vi "Update Dates.vi"(9 "date time rec":T1, 10 "Display State In":cluster{"Month":i32, "Day":i32, "Year":i32}, 11 "Dates":refnum<vi>) -> ()   [LabVIEW 2019, in "Custom Calendar.xctl"]
uses:
  Custom Calendar.xctl
panel:
  out "Month":string[][](array[string])
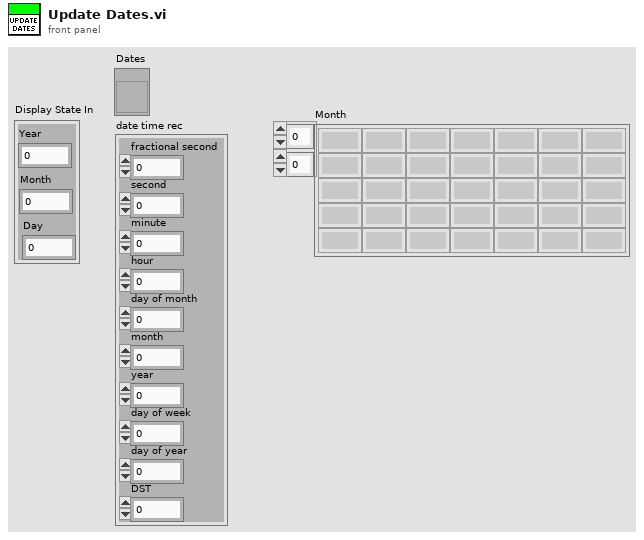
[diagram p1: front panel]
types:
  T1 = cluster{"fractional second":dbl, "second":i32, "minute":i32, "hour":i32, "day of month":i32, "month":i32, "year":i32, "day of week":i32, "day of year":i32, "DST":i32}
  T2 = typedef "LVDateTimeRec.ctl" = cluster{"fractional second":dbl, "second":i32, "minute":i32, "hour":i32, "day of month":i32, "month":i32, "year":i32, "day of week":i32, "day of year":i32, "DST":i32}
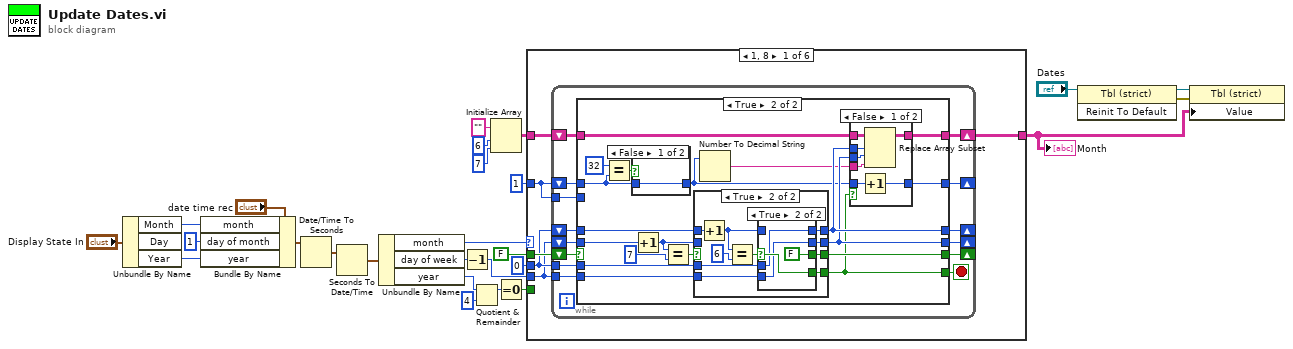
[diagram p0: block diagram]
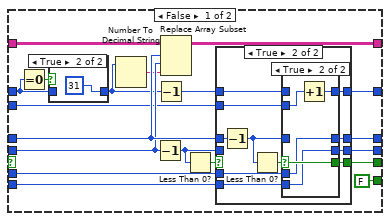
[diagram p2: hidden frame]
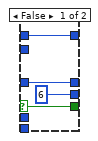
[diagram p5: hidden frame]
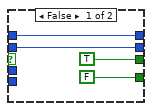
[diagram p7: hidden frame]
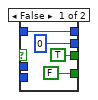
[diagram p8: hidden frame]
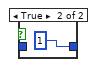
[diagram p9: hidden frame]
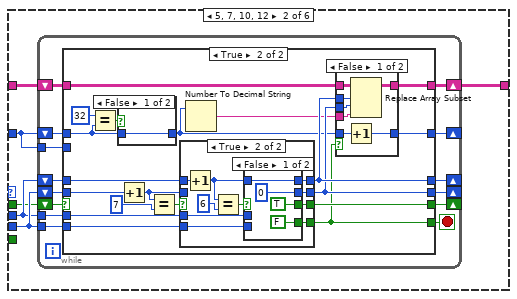
[diagram p10: hidden frame]
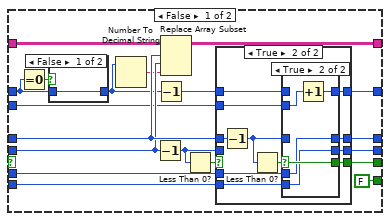
[diagram p11: hidden frame]
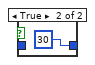
[diagram p12: hidden frame]
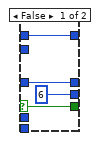
[diagram p14: hidden frame]
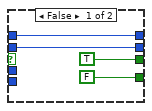
[diagram p16: hidden frame]
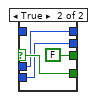
[diagram p17: hidden frame]
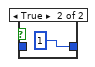
[diagram p18: hidden frame]
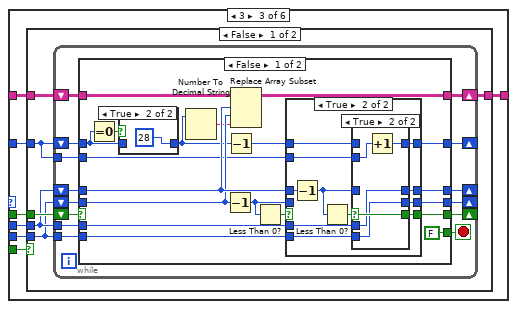
[diagram p19: hidden frame]
diagram:
  n1 = Unbundle By Name("Display State In") -> ("Month"=w14:i32, "Year"=w15:i32)  [unwired: 1 out]
  n2 = Bundle By Name(cluster="date time rec", "month"=w14, "day of month"=1, "year"=w15) -> (w26:T1)
  n3 = Date/Time To Seconds(2:w26) -> (0:w25:timestamp)  [unwired: 1 in]
  n4 = Seconds To Date/Time(time stamp (now)=w25) -> (date time rec=w23:T2)  [unwired: 1 in]
  n5 = Unbundle By Name(w23) -> ("month"=w22:i32, "day of week"=w8:i32, "year"=w20:i32)
  n6 = Decrement(x=w8) -> (x-1=w9:i32)
  n7 = Quotient & Remainder(x=w20, y=4) -> (x-y*floor(x/y)=w18:i32)  [unwired: 1 out]
  n8 = Initialize Array("", 6 ("dimension size"), 7 ("dimension size")) -> (w10:string[][])
  n9 = Equal To 0?(x=w18) -> (x = 0?=w17:bool)
  n10 = case shown="1, 8" w22 {
    tunnel: 1 ("day of month") -> [w27 w145 w265 w507 w747 _]
    tunnel: w10 -> [w32 w149 w266 w506 w748 w860]
    tunnel: [w31 w148 w261 w502 w743 w860] -> w1
    tunnel: w9 -> [w28 w147 w262 w503 w744 _]
    tunnel: 0 -> [w29 w146 w263 w504 w746 _]
    tunnel: FALSE -> [w30 w144 w264 w505 w745 _]
    tunnel: w17 -> [_ _ w267 w508 _ _]
    frame 1, 8 {
      n11 = while {
        shift-right: [w38] -> _
        shift-left: w29 -> [w46]
        shift-right: [w40] -> _
        shift-left: w28 -> [w45]
        shift-right: [w39] -> _
        shift-left: w30 -> [w34]
        shift-right: [w41] -> _
        shift-left: w27 -> [w44]
        shift-right: [w42] -> w31
        shift-left: w32 -> [w43]
        tunnel: w28 -> [w36]
        tunnel: w29 -> [w35]
        tunnel: w27 -> [w33]
        stop <- w37 stop-if-true
        n12 = case shown="True" w34 {
          tunnel: w46 -> [w64 w104]
          tunnel: w45 -> [w63 w103]
          tunnel: w44 -> [w65 w93]
          tunnel: w43 -> [w62 w109]
          tunnel: [w61 w108] -> w42
          tunnel: w36 -> [w60 w100]
          tunnel: w35 -> [w59 w101]
          tunnel: [w48 w94] -> w41
          tunnel: [w58 w98] -> w40
          tunnel: [w57 w102] -> w39
          tunnel: [w56 w99] -> w38
          tunnel: [FALSE w96] -> w37
          tunnel: w33 -> [w49 _]
          frame False {
            n13 = Equal To 0?(x=w65) -> (x = 0?=w53:bool)
            n14 = case shown="True" w53 {
              tunnel: [w66 31] -> w52
              tunnel: w65 -> [w66 _]
              frame False {
              }
              frame True {
              }
            }
            n15 = Number To Decimal String(number=w52) -> (decimal integer string=w55:string)  [unwired: 1 in]
            n16 = Decrement(x=w63) -> (x-1=w51:i32)
            n17 = Decrement(x=w52) -> (x-1=w47:i32)
            n18 = Replace Array Subset(array=w62, new element=w55, index (row)=w64, index (col)=w63) -> (w61:string[][])
            n19 = Less Than 0?(x=w51) -> (x < 0?=w54:bool)
            n20 = case shown="True" w54 {
              selector: w54 -> [w70 _]
              tunnel: w64 -> [w69 w82]
              tunnel: w59 -> [_ w79]
              tunnel: w60 -> [_ w78]
              tunnel: w51 -> [w71 _]
              tunnel: [w71 w77] -> w58
              tunnel: [w70 w76] -> w57
              tunnel: [w69 w75] -> w56
              tunnel: w49 -> [_ w72]
              tunnel: [w68 w74] -> w48
              tunnel: w47 -> [w68 w73]
              frame False {
              }
              frame True {
                n21 = Decrement(x=w82) -> (x-1=w80:i32)
                n22 = Less Than 0?(x=w80) -> (x < 0?=w81:bool)
                n23 = case shown="True" w81 {
                  selector: w81 -> [w85 w91]
                  tunnel: w80 -> [w84 _]
                  tunnel: w79 -> [_ w90]
                  tunnel: w78 -> [_ w89]
                  tunnel: [6 w89] -> w77
                  tunnel: [w85 w91] -> w76
                  tunnel: [w84 w90] -> w75
                  tunnel: w73 -> [w83 _]
                  tunnel: [w83 w88] -> w74
                  tunnel: w72 -> [_ w87]
                  frame False {
                  }
                  frame True {
                    n24 = Increment(x=w87) -> (x+1=w88:i32)
                  }
                }
              }
            }
          }
          frame True {
            n25 = Equal?(x=32 ("y"), y=w93) -> (x = y?=w110:bool)
            n26 = case shown="False" w110 {
              tunnel: [w142 1] -> w95
              tunnel: w93 -> [w142 _]
              frame False {
              }
              frame True {
              }
            }
            n27 = Increment(x=w103) -> (x+1=w105:i32)
            n28 = Equal?(x=w105, y=7) -> (x = y?=w106:bool)
            n29 = case shown="True" w106 {
              tunnel: w105 -> [w123 _]
              tunnel: w104 -> [w122 w133]
              tunnel: [w122 w129] -> w99
              tunnel: [TRUE w128] -> w102
              tunnel: [w123 w127] -> w98
              tunnel: [FALSE w126] -> w96
              tunnel: w101 -> [_ w125]
              tunnel: w100 -> [_ w124]
              frame False {
              }
              frame True {
                n30 = Increment(x=w133) -> (x+1=w130:i32)
                n31 = Equal?(x=w130, y=6) -> (x = y?=w131:bool)
                n32 = case shown="True" w131 {
                  selector: w131 -> [_ w141]
                  tunnel: w130 -> [w137 _]
                  tunnel: [w137 w140] -> w129
                  tunnel: [TRUE FALSE] -> w128
                  tunnel: [0 ("y") w139] -> w127
                  tunnel: [FALSE w141] -> w126
                  tunnel: w125 -> [_ w140]
                  tunnel: w124 -> [_ w139]
                  frame False {
                  }
                  frame True {
                  }
                }
              }
            }
            n33 = Number To Decimal String(number=w95) -> (decimal integer string=w97:string)  [unwired: 1 in]
            n34 = case shown="False" w96 {
              tunnel: w109 -> [w117 w119]
              tunnel: [w116 w119] -> w108
              tunnel: w99 -> [w115 _]
              tunnel: w98 -> [w114 _]
              tunnel: w97 -> [w113 _]
              tunnel: w95 -> [w112 w118]
              tunnel: [w111 w118] -> w94
              frame False {
                n35 = Increment(x=w112) -> (x+1=w111:i32)
                n36 = Replace Array Subset(array=w117, new element=w113, index (row)=w115, index (col)=w114) -> (w116:string[][])
              }
              frame True {
              }
            }
          }
        }
      }
    }
    frame 5, 7, 10, 12 {
      n37 = while {
        shift-right: [w155] -> _
        shift-left: w146 -> [w163]
        shift-right: [w157] -> _
        shift-left: w147 -> [w162]
        shift-right: [w156] -> _
        shift-left: w144 -> [w151]
        shift-right: [w158] -> _
        shift-left: w145 -> [w161]
        shift-right: [w159] -> w148
        shift-left: w149 -> [w160]
        tunnel: w147 -> [w153]
        tunnel: w146 -> [w152]
        tunnel: w145 -> [w150]
        stop <- w154 stop-if-true
        n38 = case shown="True" w151 {
          tunnel: w163 -> [w181 w221]
          tunnel: w162 -> [w180 w220]
          tunnel: w161 -> [w182 w210]
          tunnel: w160 -> [w179 w226]
          tunnel: [w178 w225] -> w159
          tunnel: w153 -> [w177 w217]
          tunnel: w152 -> [w176 w218]
          tunnel: [w165 w211] -> w158
          tunnel: [w175 w215] -> w157
          tunnel: [w174 w219] -> w156
          tunnel: [w173 w216] -> w155
          tunnel: [FALSE w213] -> w154
          tunnel: w150 -> [w166 _]
          frame False {
            n39 = Equal To 0?(x=w182) -> (x = 0?=w170:bool)
            n40 = case shown="False" w170 {
              tunnel: [w183 30] -> w169
              tunnel: w182 -> [w183 _]
              frame False {
              }
              frame True {
              }
            }
            n41 = Number To Decimal String(number=w169) -> (decimal integer string=w172:string)  [unwired: 1 in]
            n42 = Decrement(x=w180) -> (x-1=w168:i32)
            n43 = Decrement(x=w169) -> (x-1=w164:i32)
            n44 = Replace Array Subset(array=w179, new element=w172, index (row)=w181, index (col)=w180) -> (w178:string[][])
            n45 = Less Than 0?(x=w168) -> (x < 0?=w171:bool)
            n46 = case shown="True" w171 {
              selector: w171 -> [w187 _]
              tunnel: w181 -> [w186 w199]
              tunnel: w176 -> [_ w196]
              tunnel: w177 -> [_ w195]
              tunnel: w168 -> [w188 _]
              tunnel: [w188 w194] -> w175
              tunnel: [w187 w193] -> w174
              tunnel: [w186 w192] -> w173
              tunnel: w166 -> [_ w189]
              tunnel: [w185 w191] -> w165
              tunnel: w164 -> [w185 w190]
              frame False {
              }
              frame True {
                n47 = Decrement(x=w199) -> (x-1=w197:i32)
                n48 = Less Than 0?(x=w197) -> (x < 0?=w198:bool)
                n49 = case shown="True" w198 {
                  selector: w198 -> [w202 w208]
                  tunnel: w197 -> [w201 _]
                  tunnel: w196 -> [_ w207]
                  tunnel: w195 -> [_ w206]
                  tunnel: [6 w206] -> w194
                  tunnel: [w202 w208] -> w193
                  tunnel: [w201 w207] -> w192
                  tunnel: w190 -> [w200 _]
                  tunnel: [w200 w205] -> w191
                  tunnel: w189 -> [_ w204]
                  frame False {
                  }
                  frame True {
                    n50 = Increment(x=w204) -> (x+1=w205:i32)
                  }
                }
              }
            }
          }
          frame True {
            n51 = Equal?(x=32 ("y"), y=w210) -> (x = y?=w227:bool)
            n52 = case shown="False" w227 {
              tunnel: [w259 1] -> w212
              tunnel: w210 -> [w259 _]
              frame False {
              }
              frame True {
              }
            }
            n53 = Increment(x=w220) -> (x+1=w222:i32)
            n54 = Equal?(x=w222, y=7) -> (x = y?=w223:bool)
            n55 = case shown="True" w223 {
              tunnel: w222 -> [w240 _]
              tunnel: w221 -> [w239 w250]
              tunnel: [w239 w246] -> w216
              tunnel: [TRUE w245] -> w219
              tunnel: [w240 w244] -> w215
              tunnel: [FALSE w243] -> w213
              tunnel: w218 -> [_ w242]
              tunnel: w217 -> [_ w241]
              frame False {
              }
              frame True {
                n56 = Increment(x=w250) -> (x+1=w247:i32)
                n57 = Equal?(x=w247, y=6) -> (x = y?=w248:bool)
                n58 = case shown="False" w248 {
                  selector: w248 -> [_ w258]
                  tunnel: w247 -> [w254 _]
                  tunnel: [w254 w257] -> w246
                  tunnel: [TRUE FALSE] -> w245
                  tunnel: [0 ("y") w256] -> w244
                  tunnel: [FALSE w258] -> w243
                  tunnel: w242 -> [_ w257]
                  tunnel: w241 -> [_ w256]
                  frame False {
                  }
                  frame True {
                  }
                }
              }
            }
            n59 = Number To Decimal String(number=w212) -> (decimal integer string=w214:string)  [unwired: 1 in]
            n60 = case shown="False" w213 {
              tunnel: w226 -> [w234 w236]
              tunnel: [w233 w236] -> w225
              tunnel: w216 -> [w232 _]
              tunnel: w215 -> [w231 _]
              tunnel: w214 -> [w230 _]
              tunnel: w212 -> [w229 w235]
              tunnel: [w228 w235] -> w211
              frame False {
                n61 = Increment(x=w229) -> (x+1=w228:i32)
                n62 = Replace Array Subset(array=w234, new element=w230, index (row)=w232, index (col)=w231) -> (w233:string[][])
              }
              frame True {
              }
            }
          }
        }
      }
    }
    frame 3 {
      n63 = case shown="False" w267 {
        tunnel: w266 -> [w269 w390]
        tunnel: w265 -> [w270 w389]
        tunnel: w264 -> [w273 w388]
        tunnel: w263 -> [w272 w387]
        tunnel: w262 -> [w271 w386]
        tunnel: [w268 w385] -> w261
        frame False {
          n64 = while {
            shift-right: [w279] -> _
            shift-left: w272 -> [w287]
            shift-right: [w281] -> _
            shift-left: w271 -> [w286]
            shift-right: [w280] -> _
            shift-left: w273 -> [w275]
            shift-right: [w282] -> _
            shift-left: w270 -> [w285]
            shift-right: [w283] -> w268
            shift-left: w269 -> [w284]
            tunnel: w271 -> [w277]
            tunnel: w272 -> [w276]
            tunnel: w270 -> [w274]
            stop <- w278 stop-if-true
            n65 = case shown="False" w275 {
              tunnel: w287 -> [w305 w345]
              tunnel: w286 -> [w304 w344]
              tunnel: w285 -> [w306 w334]
              tunnel: w284 -> [w303 w350]
              tunnel: [w302 w349] -> w283
              tunnel: w277 -> [w301 w341]
              tunnel: w276 -> [w300 w342]
              tunnel: [w289 w335] -> w282
              tunnel: [w299 w339] -> w281
              tunnel: [w298 w343] -> w280
              tunnel: [w297 w340] -> w279
              tunnel: [FALSE w337] -> w278
              tunnel: w274 -> [w290 _]
              frame False {
                n66 = Equal To 0?(x=w306) -> (x = 0?=w294:bool)
                n67 = case shown="True" w294 {
                  tunnel: [w307 28] -> w293
                  tunnel: w306 -> [w307 _]
                  frame False {
                  }
                  frame True {
                  }
                }
                n68 = Number To Decimal String(number=w293) -> (decimal integer string=w296:string)  [unwired: 1 in]
                n69 = Decrement(x=w304) -> (x-1=w292:i32)
                n70 = Decrement(x=w293) -> (x-1=w288:i32)
                n71 = Replace Array Subset(array=w303, new element=w296, index (row)=w305, index (col)=w304) -> (w302:string[][])
                n72 = Less Than 0?(x=w292) -> (x < 0?=w295:bool)
                n73 = case shown="True" w295 {
                  selector: w295 -> [w311 _]
                  tunnel: w305 -> [w310 w323]
                  tunnel: w300 -> [_ w320]
                  tunnel: w301 -> [_ w319]
                  tunnel: w292 -> [w312 _]
                  tunnel: [w312 w318] -> w299
                  tunnel: [w311 w317] -> w298
                  tunnel: [w310 w316] -> w297
                  tunnel: w290 -> [_ w313]
                  tunnel: [w309 w315] -> w289
                  tunnel: w288 -> [w309 w314]
                  frame False {
                  }
                  frame True {
                    n74 = Decrement(x=w323) -> (x-1=w321:i32)
                    n75 = Less Than 0?(x=w321) -> (x < 0?=w322:bool)
                    n76 = case shown="True" w322 {
                      selector: w322 -> [w326 w332]
                      tunnel: w321 -> [w325 _]
                      tunnel: w320 -> [_ w331]
                      tunnel: w319 -> [_ w330]
                      tunnel: [6 w330] -> w318
                      tunnel: [w326 w332] -> w317
                      tunnel: [w325 w331] -> w316
                      tunnel: w314 -> [w324 _]
                      tunnel: [w324 w329] -> w315
                      tunnel: w313 -> [_ w328]
                      frame False {
                      }
                      frame True {
                        n77 = Increment(x=w328) -> (x+1=w329:i32)
                      }
                    }
                  }
                }
              }
              frame True {
                n78 = Equal?(x=32 ("y"), y=w334) -> (x = y?=w351:bool)
                n79 = case shown="True" w351 {
                  tunnel: [w383 1] -> w336
                  tunnel: w334 -> [w383 _]
                  frame False {
                  }
                  frame True {
                  }
                }
                n80 = Increment(x=w344) -> (x+1=w346:i32)
                n81 = Equal?(x=w346, y=7) -> (x = y?=w347:bool)
                n82 = case shown="True" w347 {
                  tunnel: w346 -> [w364 _]
                  tunnel: w345 -> [w363 w374]
                  tunnel: [w363 w370] -> w340
                  tunnel: [TRUE w369] -> w343
                  tunnel: [w364 w368] -> w339
                  tunnel: [FALSE w367] -> w337
                  tunnel: w342 -> [_ w366]
                  tunnel: w341 -> [_ w365]
                  frame False {
                  }
                  frame True {
                    n83 = Increment(x=w374) -> (x+1=w371:i32)
                    n84 = Equal?(x=w371, y=6) -> (x = y?=w372:bool)
                    n85 = case shown="False" w372 {
                      selector: w372 -> [_ w382]
                      tunnel: w371 -> [w378 _]
                      tunnel: [w378 w381] -> w370
                      tunnel: [TRUE FALSE] -> w369
                      tunnel: [0 ("y") w380] -> w368
                      tunnel: [FALSE w382] -> w367
                      tunnel: w366 -> [_ w381]
                      tunnel: w365 -> [_ w380]
                      frame False {
                      }
                      frame True {
                      }
                    }
                  }
                }
                n86 = Number To Decimal String(number=w336) -> (decimal integer string=w338:string)  [unwired: 1 in]
                n87 = case shown="False" w337 {
                  tunnel: w350 -> [w358 w360]
                  tunnel: [w357 w360] -> w349
                  tunnel: w340 -> [w356 _]
                  tunnel: w339 -> [w355 _]
                  tunnel: w338 -> [w354 _]
                  tunnel: w336 -> [w353 w359]
                  tunnel: [w352 w359] -> w335
                  frame False {
                    n88 = Increment(x=w353) -> (x+1=w352:i32)
                    n89 = Replace Array Subset(array=w358, new element=w354, index (row)=w356, index (col)=w355) -> (w357:string[][])
                  }
                  frame True {
                  }
                }
              }
            }
          }
        }
        frame True {
          n90 = while {
            shift-right: [w396] -> _
            shift-left: w387 -> [w404]
            shift-right: [w398] -> _
            shift-left: w386 -> [w403]
            shift-right: [w397] -> _
            shift-left: w388 -> [w392]
            shift-right: [w399] -> _
            shift-left: w389 -> [w402]
            shift-right: [w400] -> w385
            shift-left: w390 -> [w401]
            tunnel: w386 -> [w394]
            tunnel: w387 -> [w393]
            tunnel: w389 -> [w391]
            stop <- w395 stop-if-true
            n91 = case shown="False" w392 {
              tunnel: w404 -> [w422 w462]
              tunnel: w403 -> [w421 w461]
              tunnel: w402 -> [w423 w451]
              tunnel: w401 -> [w420 w467]
              tunnel: [w419 w466] -> w400
              tunnel: w394 -> [w418 w458]
              tunnel: w393 -> [w417 w459]
              tunnel: [w406 w452] -> w399
              tunnel: [w416 w456] -> w398
              tunnel: [w415 w460] -> w397
              tunnel: [w414 w457] -> w396
              tunnel: [FALSE w454] -> w395
              tunnel: w391 -> [w407 _]
              frame False {
                n92 = Equal To 0?(x=w423) -> (x = 0?=w411:bool)
                n93 = case shown="True" w411 {
                  tunnel: [w424 29] -> w410
                  tunnel: w423 -> [w424 _]
                  frame False {
                  }
                  frame True {
                  }
                }
                n94 = Number To Decimal String(number=w410) -> (decimal integer string=w413:string)  [unwired: 1 in]
                n95 = Decrement(x=w421) -> (x-1=w409:i32)
                n96 = Decrement(x=w410) -> (x-1=w405:i32)
                n97 = Replace Array Subset(array=w420, new element=w413, index (row)=w422, index (col)=w421) -> (w419:string[][])
                n98 = Less Than 0?(x=w409) -> (x < 0?=w412:bool)
                n99 = case shown="True" w412 {
                  selector: w412 -> [w428 _]
                  tunnel: w422 -> [w427 w440]
                  tunnel: w417 -> [_ w437]
                  tunnel: w418 -> [_ w436]
                  tunnel: w409 -> [w429 _]
                  tunnel: [w429 w435] -> w416
                  tunnel: [w428 w434] -> w415
                  tunnel: [w427 w433] -> w414
                  tunnel: w407 -> [_ w430]
                  tunnel: [w426 w432] -> w406
                  tunnel: w405 -> [w426 w431]
                  frame False {
                  }
                  frame True {
                    n100 = Decrement(x=w440) -> (x-1=w438:i32)
                    n101 = Less Than 0?(x=w438) -> (x < 0?=w439:bool)
                    n102 = case shown="True" w439 {
                      selector: w439 -> [w443 w449]
                      tunnel: w438 -> [w442 _]
                      tunnel: w437 -> [_ w448]
                      tunnel: w436 -> [_ w447]
                      tunnel: [6 w447] -> w435
                      tunnel: [w443 w449] -> w434
                      tunnel: [w442 w448] -> w433
                      tunnel: w431 -> [w441 _]
                      tunnel: [w441 w446] -> w432
                      tunnel: w430 -> [_ w445]
                      frame False {
                      }
                      frame True {
                        n103 = Increment(x=w445) -> (x+1=w446:i32)
                      }
                    }
                  }
                }
              }
              frame True {
                n104 = Equal?(x=32 ("y"), y=w451) -> (x = y?=w468:bool)
                n105 = case shown="False" w468 {
                  tunnel: [w500 1] -> w453
                  tunnel: w451 -> [w500 _]
                  frame False {
                  }
                  frame True {
                  }
                }
                n106 = Increment(x=w461) -> (x+1=w463:i32)
                n107 = Equal?(x=w463, y=7) -> (x = y?=w464:bool)
                n108 = case shown="True" w464 {
                  tunnel: w463 -> [w481 _]
                  tunnel: w462 -> [w480 w491]
                  tunnel: [w480 w487] -> w457
                  tunnel: [TRUE w486] -> w460
                  tunnel: [w481 w485] -> w456
                  tunnel: [FALSE w484] -> w454
                  tunnel: w459 -> [_ w483]
                  tunnel: w458 -> [_ w482]
                  frame False {
                  }
                  frame True {
                    n109 = Increment(x=w491) -> (x+1=w488:i32)
                    n110 = Equal?(x=w488, y=6) -> (x = y?=w489:bool)
                    n111 = case shown="False" w489 {
                      selector: w489 -> [_ w499]
                      tunnel: w488 -> [w495 _]
                      tunnel: [w495 w498] -> w487
                      tunnel: [TRUE FALSE] -> w486
                      tunnel: [0 ("y") w497] -> w485
                      tunnel: [FALSE w499] -> w484
                      tunnel: w483 -> [_ w498]
                      tunnel: w482 -> [_ w497]
                      frame False {
                      }
                      frame True {
                      }
                    }
                  }
                }
                n112 = Number To Decimal String(number=w453) -> (decimal integer string=w455:string)  [unwired: 1 in]
                n113 = case shown="False" w454 {
                  tunnel: w467 -> [w475 w477]
                  tunnel: [w474 w477] -> w466
                  tunnel: w457 -> [w473 _]
                  tunnel: w456 -> [w472 _]
                  tunnel: w455 -> [w471 _]
                  tunnel: w453 -> [w470 w476]
                  tunnel: [w469 w476] -> w452
                  frame False {
                    n114 = Increment(x=w470) -> (x+1=w469:i32)
                    n115 = Replace Array Subset(array=w475, new element=w471, index (row)=w473, index (col)=w472) -> (w474:string[][])
                  }
                  frame True {
                  }
                }
              }
            }
          }
        }
      }
    }
    frame 2 {
      n116 = case shown="False" w508 {
        tunnel: w507 -> [w513 w630]
        tunnel: w506 -> [w514 w631]
        tunnel: w505 -> [w512 w629]
        tunnel: w504 -> [w511 w628]
        tunnel: w503 -> [w510 w627]
        tunnel: [w509 w626] -> w502
        frame False {
          n117 = while {
            shift-right: [w520] -> _
            shift-left: w511 -> [w528]
            shift-right: [w522] -> _
            shift-left: w510 -> [w527]
            shift-right: [w521] -> _
            shift-left: w512 -> [w516]
            shift-right: [w523] -> _
            shift-left: w513 -> [w526]
            shift-right: [w524] -> w509
            shift-left: w514 -> [w525]
            tunnel: w510 -> [w518]
            tunnel: w511 -> [w517]
            tunnel: w513 -> [w515]
            stop <- w519 stop-if-true
            n118 = case shown="True" w516 {
              tunnel: w528 -> [w546 w586]
              tunnel: w527 -> [w545 w585]
              tunnel: w526 -> [w547 w575]
              tunnel: w525 -> [w544 w591]
              tunnel: [w543 w590] -> w524
              tunnel: w518 -> [w542 w582]
              tunnel: w517 -> [w541 w583]
              tunnel: [w530 w576] -> w523
              tunnel: [w540 w580] -> w522
              tunnel: [w539 w584] -> w521
              tunnel: [w538 w581] -> w520
              tunnel: [FALSE w578] -> w519
              tunnel: w515 -> [w531 _]
              frame False {
                n119 = Equal To 0?(x=w547) -> (x = 0?=w535:bool)
                n120 = case shown="True" w535 {
                  tunnel: [w548 31] -> w534
                  tunnel: w547 -> [w548 _]
                  frame False {
                  }
                  frame True {
                  }
                }
                n121 = Number To Decimal String(number=w534) -> (decimal integer string=w537:string)  [unwired: 1 in]
                n122 = Decrement(x=w545) -> (x-1=w533:i32)
                n123 = Decrement(x=w534) -> (x-1=w529:i32)
                n124 = Replace Array Subset(array=w544, new element=w537, index (row)=w546, index (col)=w545) -> (w543:string[][])
                n125 = Less Than 0?(x=w533) -> (x < 0?=w536:bool)
                n126 = case shown="False" w536 {
                  selector: w536 -> [w552 _]
                  tunnel: w546 -> [w551 w564]
                  tunnel: w541 -> [_ w561]
                  tunnel: w542 -> [_ w560]
                  tunnel: w533 -> [w553 _]
                  tunnel: [w553 w559] -> w540
                  tunnel: [w552 w558] -> w539
                  tunnel: [w551 w557] -> w538
                  tunnel: w531 -> [_ w554]
                  tunnel: [w550 w556] -> w530
                  tunnel: w529 -> [w550 w555]
                  frame False {
                  }
                  frame True {
                    n127 = Decrement(x=w564) -> (x-1=w562:i32)
                    n128 = Less Than 0?(x=w562) -> (x < 0?=w563:bool)
                    n129 = case shown="True" w563 {
                      selector: w563 -> [w567 w573]
                      tunnel: w562 -> [w566 _]
                      tunnel: w561 -> [_ w572]
                      tunnel: w560 -> [_ w571]
                      tunnel: [6 w571] -> w559
                      tunnel: [w567 w573] -> w558
                      tunnel: [w566 w572] -> w557
                      tunnel: w555 -> [w565 _]
                      tunnel: [w565 w570] -> w556
                      tunnel: w554 -> [_ w569]
                      frame False {
                      }
                      frame True {
                        n130 = Increment(x=w569) -> (x+1=w570:i32)
                      }
                    }
                  }
                }
              }
              frame True {
                n131 = Equal?(x=28 ("y"), y=w575) -> (x = y?=w592:bool)
                n132 = case shown="True" w592 {
                  tunnel: [w624 1] -> w577
                  tunnel: w575 -> [w624 _]
                  frame False {
                  }
                  frame True {
                  }
                }
                n133 = Increment(x=w585) -> (x+1=w587:i32)
                n134 = Equal?(x=w587, y=7) -> (x = y?=w588:bool)
                n135 = case shown="True" w588 {
                  tunnel: w587 -> [w605 _]
                  tunnel: w586 -> [w604 w615]
                  tunnel: [w604 w611] -> w581
                  tunnel: [TRUE w610] -> w584
                  tunnel: [w605 w609] -> w580
                  tunnel: [FALSE w608] -> w578
                  tunnel: w583 -> [_ w607]
                  tunnel: w582 -> [_ w606]
                  frame False {
                  }
                  frame True {
                    n136 = Increment(x=w615) -> (x+1=w612:i32)
                    n137 = Equal?(x=w612, y=6) -> (x = y?=w613:bool)
                    n138 = case shown="True" w613 {
                      selector: w613 -> [_ w623]
                      tunnel: w612 -> [w619 _]
                      tunnel: [w619 w622] -> w611
                      tunnel: [TRUE FALSE] -> w610
                      tunnel: [0 ("y") w621] -> w609
                      tunnel: [FALSE w623] -> w608
                      tunnel: w607 -> [_ w622]
                      tunnel: w606 -> [_ w621]
                      frame False {
                      }
                      frame True {
                      }
                    }
                  }
                }
                n139 = Number To Decimal String(number=w577) -> (decimal integer string=w579:string)  [unwired: 1 in]
                n140 = case shown="False" w578 {
                  tunnel: w591 -> [w599 w601]
                  tunnel: [w598 w601] -> w590
                  tunnel: w581 -> [w597 _]
                  tunnel: w580 -> [w596 _]
                  tunnel: w579 -> [w595 _]
                  tunnel: w577 -> [w594 w600]
                  tunnel: [w593 w600] -> w576
                  frame False {
                    n141 = Increment(x=w594) -> (x+1=w593:i32)
                    n142 = Replace Array Subset(array=w599, new element=w595, index (row)=w597, index (col)=w596) -> (w598:string[][])
                  }
                  frame True {
                  }
                }
              }
            }
          }
        }
        frame True {
          n143 = while {
            shift-right: [w637] -> _
            shift-left: w628 -> [w645]
            shift-right: [w639] -> _
            shift-left: w627 -> [w644]
            shift-right: [w638] -> _
            shift-left: w629 -> [w633]
            shift-right: [w640] -> _
            shift-left: w630 -> [w643]
            shift-right: [w641] -> w626
            shift-left: w631 -> [w642]
            tunnel: w627 -> [w635]
            tunnel: w628 -> [w634]
            tunnel: w630 -> [w632]
            stop <- w636 stop-if-true
            n144 = case shown="True" w633 {
              tunnel: w645 -> [w663 w703]
              tunnel: w644 -> [w662 w702]
              tunnel: w643 -> [w664 w692]
              tunnel: w642 -> [w661 w708]
              tunnel: [w660 w707] -> w641
              tunnel: w635 -> [w659 w699]
              tunnel: w634 -> [w658 w700]
              tunnel: [w647 w693] -> w640
              tunnel: [w657 w697] -> w639
              tunnel: [w656 w701] -> w638
              tunnel: [w655 w698] -> w637
              tunnel: [FALSE w695] -> w636
              tunnel: w632 -> [w648 _]
              frame False {
                n145 = Equal To 0?(x=w664) -> (x = 0?=w652:bool)
                n146 = case shown="True" w652 {
                  tunnel: [w665 31] -> w651
                  tunnel: w664 -> [w665 _]
                  frame False {
                  }
                  frame True {
                  }
                }
                n147 = Number To Decimal String(number=w651) -> (decimal integer string=w654:string)  [unwired: 1 in]
                n148 = Decrement(x=w662) -> (x-1=w650:i32)
                n149 = Decrement(x=w651) -> (x-1=w646:i32)
                n150 = Replace Array Subset(array=w661, new element=w654, index (row)=w663, index (col)=w662) -> (w660:string[][])
                n151 = Less Than 0?(x=w650) -> (x < 0?=w653:bool)
                n152 = case shown="True" w653 {
                  selector: w653 -> [w669 _]
                  tunnel: w663 -> [w668 w681]
                  tunnel: w658 -> [_ w678]
                  tunnel: w659 -> [_ w677]
                  tunnel: w650 -> [w670 _]
                  tunnel: [w670 w676] -> w657
                  tunnel: [w669 w675] -> w656
                  tunnel: [w668 w674] -> w655
                  tunnel: w648 -> [_ w671]
                  tunnel: [w667 w673] -> w647
                  tunnel: w646 -> [w667 w672]
                  frame False {
                  }
                  frame True {
                    n153 = Decrement(x=w681) -> (x-1=w679:i32)
                    n154 = Less Than 0?(x=w679) -> (x < 0?=w680:bool)
                    n155 = case shown="True" w680 {
                      selector: w680 -> [w684 w690]
                      tunnel: w679 -> [w683 _]
                      tunnel: w678 -> [_ w689]
                      tunnel: w677 -> [_ w688]
                      tunnel: [6 w688] -> w676
                      tunnel: [w684 w690] -> w675
                      tunnel: [w683 w689] -> w674
                      tunnel: w672 -> [w682 _]
                      tunnel: [w682 w687] -> w673
                      tunnel: w671 -> [_ w686]
                      frame False {
                      }
                      frame True {
                        n156 = Increment(x=w686) -> (x+1=w687:i32)
                      }
                    }
                  }
                }
              }
              frame True {
                n157 = Equal?(x=29 ("y"), y=w692) -> (x = y?=w709:bool)
                n158 = case shown="True" w709 {
                  tunnel: [w741 1] -> w694
                  tunnel: w692 -> [w741 _]
                  frame False {
                  }
                  frame True {
                  }
                }
                n159 = Increment(x=w702) -> (x+1=w704:i32)
                n160 = Equal?(x=w704, y=7) -> (x = y?=w705:bool)
                n161 = case shown="True" w705 {
                  tunnel: w704 -> [w722 _]
                  tunnel: w703 -> [w721 w732]
                  tunnel: [w721 w728] -> w698
                  tunnel: [TRUE w727] -> w701
                  tunnel: [w722 w726] -> w697
                  tunnel: [FALSE w725] -> w695
                  tunnel: w700 -> [_ w724]
                  tunnel: w699 -> [_ w723]
                  frame False {
                  }
                  frame True {
                    n162 = Increment(x=w732) -> (x+1=w729:i32)
                    n163 = Equal?(x=w729, y=6) -> (x = y?=w730:bool)
                    n164 = case shown="True" w730 {
                      selector: w730 -> [_ w740]
                      tunnel: w729 -> [w736 _]
                      tunnel: [w736 w739] -> w728
                      tunnel: [TRUE FALSE] -> w727
                      tunnel: [0 ("y") w738] -> w726
                      tunnel: [FALSE w740] -> w725
                      tunnel: w724 -> [_ w739]
                      tunnel: w723 -> [_ w738]
                      frame False {
                      }
                      frame True {
                      }
                    }
                  }
                }
                n165 = Number To Decimal String(number=w694) -> (decimal integer string=w696:string)  [unwired: 1 in]
                n166 = case shown="False" w695 {
                  tunnel: w708 -> [w716 w718]
                  tunnel: [w715 w718] -> w707
                  tunnel: w698 -> [w714 _]
                  tunnel: w697 -> [w713 _]
                  tunnel: w696 -> [w712 _]
                  tunnel: w694 -> [w711 w717]
                  tunnel: [w710 w717] -> w693
                  frame False {
                    n167 = Increment(x=w711) -> (x+1=w710:i32)
                    n168 = Replace Array Subset(array=w716, new element=w712, index (row)=w714, index (col)=w713) -> (w715:string[][])
                  }
                  frame True {
                  }
                }
              }
            }
          }
        }
      }
    }
    frame 4, 6, 9, 11 {
      n169 = while {
        shift-right: [w754] -> _
        shift-left: w746 -> [w762]
        shift-right: [w756] -> _
        shift-left: w744 -> [w761]
        shift-right: [w755] -> _
        shift-left: w745 -> [w750]
        shift-right: [w757] -> _
        shift-left: w747 -> [w760]
        shift-right: [w758] -> w743
        shift-left: w748 -> [w759]
        tunnel: w744 -> [w752]
        tunnel: w746 -> [w751]
        tunnel: w747 -> [w749]
        stop <- w753 stop-if-true
        n170 = case shown="False" w750 {
          tunnel: w762 -> [w780 w820]
          tunnel: w761 -> [w779 w819]
          tunnel: w760 -> [w781 w809]
          tunnel: w759 -> [w778 w825]
          tunnel: [w777 w824] -> w758
          tunnel: w752 -> [w776 w816]
          tunnel: w751 -> [w775 w817]
          tunnel: [w764 w810] -> w757
          tunnel: [w774 w814] -> w756
          tunnel: [w773 w818] -> w755
          tunnel: [w772 w815] -> w754
          tunnel: [FALSE w812] -> w753
          tunnel: w749 -> [w765 _]
          frame False {
            n171 = Equal To 0?(x=w781) -> (x = 0?=w769:bool)
            n172 = case shown="True" w769 {
              tunnel: [w782 31] -> w768
              tunnel: w781 -> [w782 _]
              frame False {
              }
              frame True {
              }
            }
            n173 = Number To Decimal String(number=w768) -> (decimal integer string=w771:string)  [unwired: 1 in]
            n174 = Decrement(x=w779) -> (x-1=w767:i32)
            n175 = Decrement(x=w768) -> (x-1=w763:i32)
            n176 = Replace Array Subset(array=w778, new element=w771, index (row)=w780, index (col)=w779) -> (w777:string[][])
            n177 = Less Than 0?(x=w767) -> (x < 0?=w770:bool)
            n178 = case shown="True" w770 {
              selector: w770 -> [w786 _]
              tunnel: w780 -> [w785 w798]
              tunnel: w775 -> [_ w795]
              tunnel: w776 -> [_ w794]
              tunnel: w767 -> [w787 _]
              tunnel: [w787 w793] -> w774
              tunnel: [w786 w792] -> w773
              tunnel: [w785 w791] -> w772
              tunnel: w765 -> [_ w788]
              tunnel: [w784 w790] -> w764
              tunnel: w763 -> [w784 w789]
              frame False {
              }
              frame True {
                n179 = Decrement(x=w798) -> (x-1=w796:i32)
                n180 = Less Than 0?(x=w796) -> (x < 0?=w797:bool)
                n181 = case shown="True" w797 {
                  selector: w797 -> [w801 w807]
                  tunnel: w796 -> [w800 _]
                  tunnel: w795 -> [_ w806]
                  tunnel: w794 -> [_ w805]
                  tunnel: [6 w805] -> w793
                  tunnel: [w801 w807] -> w792
                  tunnel: [w800 w806] -> w791
                  tunnel: w789 -> [w799 _]
                  tunnel: [w799 w804] -> w790
                  tunnel: w788 -> [_ w803]
                  frame False {
                  }
                  frame True {
                    n182 = Increment(x=w803) -> (x+1=w804:i32)
                  }
                }
              }
            }
          }
          frame True {
            n183 = Equal?(x=31 ("y"), y=w809) -> (x = y?=w826:bool)
            n184 = case shown="True" w826 {
              tunnel: [w858 1] -> w811
              tunnel: w809 -> [w858 _]
              frame False {
              }
              frame True {
              }
            }
            n185 = Increment(x=w819) -> (x+1=w821:i32)
            n186 = Equal?(x=w821, y=7) -> (x = y?=w822:bool)
            n187 = case shown="True" w822 {
              tunnel: w821 -> [w839 _]
              tunnel: w820 -> [w838 w849]
              tunnel: [w838 w845] -> w815
              tunnel: [TRUE w844] -> w818
              tunnel: [w839 w843] -> w814
              tunnel: [FALSE w842] -> w812
              tunnel: w817 -> [_ w841]
              tunnel: w816 -> [_ w840]
              frame False {
              }
              frame True {
                n188 = Increment(x=w849) -> (x+1=w846:i32)
                n189 = Equal?(x=w846, y=6) -> (x = y?=w847:bool)
                n190 = case shown="False" w847 {
                  selector: w847 -> [_ w857]
                  tunnel: w846 -> [w853 _]
                  tunnel: [w853 w856] -> w845
                  tunnel: [TRUE FALSE] -> w844
                  tunnel: [0 ("y") w855] -> w843
                  tunnel: [FALSE w857] -> w842
                  tunnel: w841 -> [_ w856]
                  tunnel: w840 -> [_ w855]
                  frame False {
                  }
                  frame True {
                  }
                }
              }
            }
            n191 = Number To Decimal String(number=w811) -> (decimal integer string=w813:string)  [unwired: 1 in]
            n192 = case shown="False" w812 {
              tunnel: w825 -> [w833 w835]
              tunnel: [w832 w835] -> w824
              tunnel: w815 -> [w831 _]
              tunnel: w814 -> [w830 _]
              tunnel: w813 -> [w829 _]
              tunnel: w811 -> [w828 w834]
              tunnel: [w827 w834] -> w810
              frame False {
                n193 = Increment(x=w828) -> (x+1=w827:i32)
                n194 = Replace Array Subset(array=w833, new element=w829, index (row)=w831, index (col)=w830) -> (w832:string[][])
              }
              frame True {
              }
            }
          }
        }
      }
    }
    frame Default {
    }
  }
  "Month" <- w1
  n195 = invoke class="Tbl (strict)" method="Reinit To Default"(reference="Dates") -> (reference out=w3:refnum<vi>, error out=w2:errorcluster)  [unwired: 2 in, 1 out]
  n196 = property class="Tbl (strict)"(reference=w3, error in=w2, "Value"=w1) -> ()  [unwired: 2 out]
